vi "colorClassification.vi"(8 "error in":errorcluster) -> (0 "error out":errorcluster, 1 "cube color":string, 2 "object color":string)   [LabVIEW 2018]
panel:
  out "Image Out":T1(plugin-control)
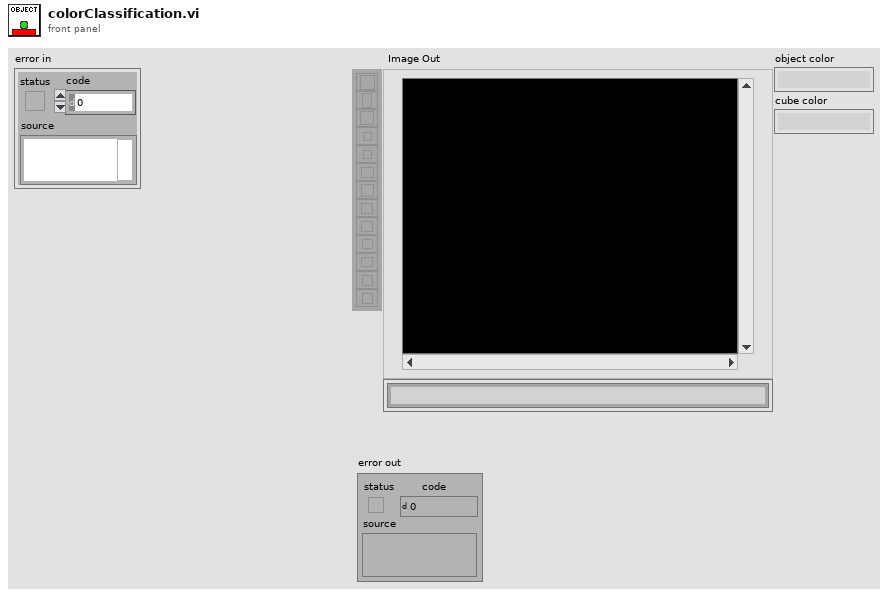
[diagram p1: front panel]
types:
  T1 = typedef "IMAQ Image.ctl" = refnum<image>
  T2 = cluster{"Global Rectangle":i32[], "Contours":cluster{"ID":enum32{"External", "Internal"}, "Type":u32, "Coordinates":i32[]}[]}
  T3 = cluster{"ID":enum32{"External", "Internal"}, "Type":u32, "Coordinates":i32[]}[]
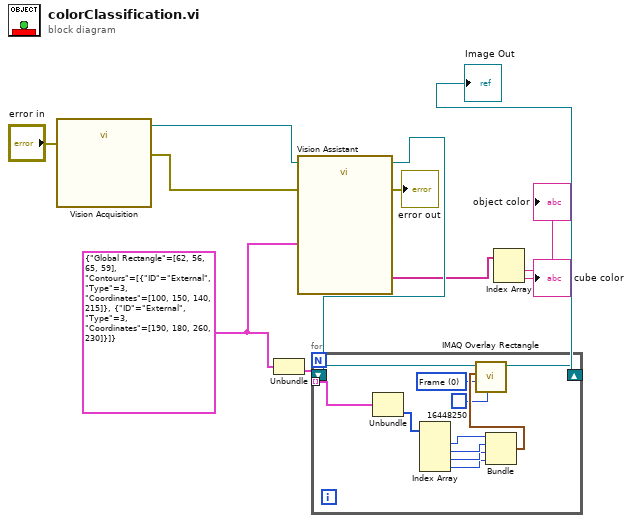
[diagram p0: block diagram]
diagram:
  w7 = T2 {"Global Rectangle"=[62, 56, 65, 59], "Contours"=[{"ID"=enum."External", "Type"=3, "Coordinates"=[100, 150, 140, 215]}, {"ID"=enum."External", "Type"=3, "Coordinates"=[190, 180, 260, 230]}]} ("ROI Descriptor (Color Classification 1)")
  n1 = call "Vision Acquisition"("error in"="error in") -> ("Image Out"=w11:T1, "error out"=w10:errorcluster)  [unwired: 25 in]
  n2 = Unbundle(w7) -> ("Contours"=w6:T3)  [unwired: 1 out]
  n3 = call "Vision Assistant"("Image In"=w11, "ROI Descriptor (Color Classification 1)"=w7, "error in"=w10) -> ("Image Out"=w5:T1, "Classes (Color Classification 1)"=w3:string[], "error out"=→"error out":errorcluster)  [unwired: 21 in, 1 out]
  n4 = for {
    tunnel: w6 -> [w12] mode=indexing
    shift-right: [w15] -> w4
    shift-left: w5 -> [w16]
    w13 = u32 0 items=["Frame", "Fill", "Highlight"] ("Drawing Mode (Frame)")
    n5 = Unbundle(w12) -> ("Coordinates"=w22:i32[])  [unwired: 2 out]
    n6 = Index Array(array=w22) -> (element #1=w21:i32, element #2=w20:i32, element #3=w19:i32, element #4=w18:i32)  [unwired: 4 in]
    n7 = Bundle(w21, w20, w19, w18) -> (w17:cluster{i32, i32, i32, i32})  [unwired: 1 in]
    n8 = call "IMAQ Overlay Rectangle"("Color"=u32 16448250, "Drawing Mode (Frame)"=w13, "Rectangle"=w17, "Image"=w16) -> ("Image Out"=w15:T1)  [unwired: 6 in, 1 out]
  }
  "Image Out" <- w4
  n9 = Index Array(array=w3) -> (element #1=→"object color":string, element #2=→"cube color":string)  [unwired: 2 in]
